vi "To Dynamic Signal.vi"(8 "error in (no error)":errorcluster, 11 "Software Lock-in in":refnum<class "Software Lock-in.lvclass">) -> (0 "error out":errorcluster, 1 "Channel names":string[](array[string]), 2 "Signal":dynamicdata(graph), 3 "Software Lock-in out":refnum<class "Software Lock-in.lvclass">, 4 "Time axis":dbl[](array[numeric]), 5 "dt":dbl)   [LabVIEW 2016, in "Software Lock-in.lvclass"]
uses:
  Software Lock-in.lvclass
  Software Lock-in.lvclass/Software Lock-in.ctl
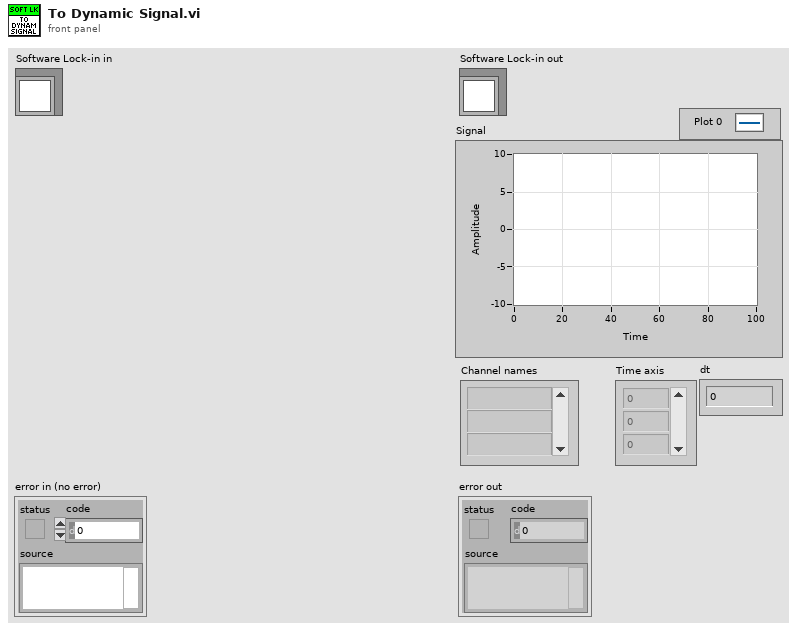
[diagram p1: front panel]
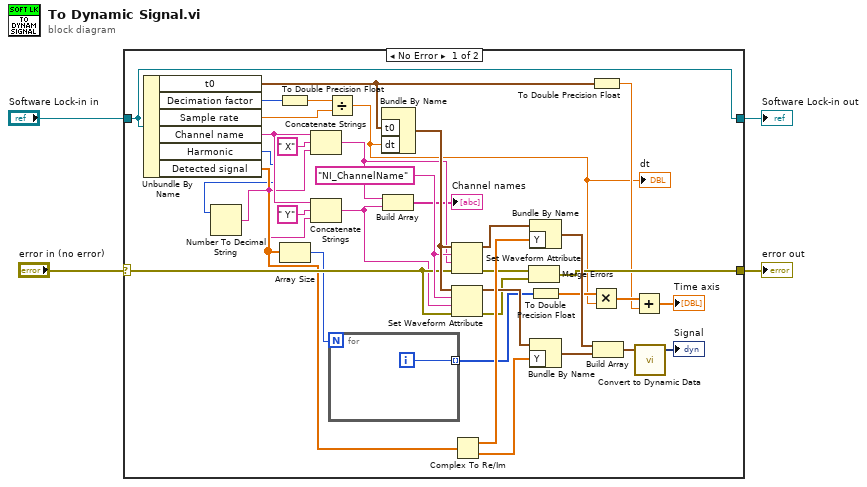
[diagram p0: block diagram]
diagram:
  n1 = case shown="No Error" "error in (no error)" {
    selector: "error in (no error)" -> [w20 w42]
    tunnel: [w19 w42] -> w3
    tunnel: [w39 w41] -> w1
    tunnel: "Software Lock-in in" -> [w39 w41]
    frame No Error {
      w33 = "NI_ChannelName" ("Channel Name")
      n2 = Unbundle By Name(w39) -> ("t0"=w10:timestamp, "Decimation factor"=w38:i32, "Sample rate"=w36:dbl, "Channel name"=w31:string, "Harmonic"=w6:i32, "Detected signal"=w15:cdb[])
      n3 = Number To Decimal String(number=w6) -> (decimal integer string=w5:string)  [unwired: 1 in]
      n4 = To Double Precision Float(number=w38) -> (double precision float=w37:dbl)
      n5 = Array Size(array=w15) -> (size(s)=w14:i32)
      n6 = Concatenate Strings(w31, " X" ("string"), w5) -> (w18:string)
      n7 = Concatenate Strings(w31, " Y" ("string"), w5) -> (w17:string)
      n8 = Divide(x=w37, y=w36) -> (x/y=w7:dbl)
      "dt" <- w7
      n9 = for {
        N: w14 -> [_]
        tunnel: [w40] -> w13 mode=indexing
        i -> [w40]
      }
      n10 = Bundle By Name("t0"=w10, "dt"=w7) -> (w34:waveform(dbl))  [unwired: 1 in]
      n11 = Build Array(w18, w17) -> (→"Channel names":string[])
      n12 = Set Waveform Attribute(4:w20, 5:w18, 6:w33, 7:w34) -> (0:w22:errorcluster, 3:w30:waveform(dbl))  [unwired: 1 out]
      n13 = Set Waveform Attribute(4:w20, 5:w17, 6:w33, 7:w34) -> (0:w21:errorcluster, 3:w28:waveform(dbl))  [unwired: 1 out]
      n14 = Complex To Re/Im(x + iy=w15) -> (x=w29:dbl[], y=w27:dbl[])
      n15 = Merge Errors(w22, w21) -> (w19:errorcluster)
      n16 = Bundle By Name(cluster=w30, "Y"=w29) -> (w26:waveform(dbl))
      n17 = Bundle By Name(cluster=w28, "Y"=w27) -> (w25:waveform(dbl))
      n18 = To Double Precision Float(number=w13) -> (double precision float=w12:dbl[])
      n19 = Multiply(x=w12, y=w7) -> (x*y=w11:dbl[])
      n20 = To Double Precision Float(number=w10) -> (double precision float=w9:dbl)
      n21 = Build Array(w26, w25) -> (w24:waveform(dbl)[])
      n22 = Add(x=w11, y=w9) -> (x+y=→"Time axis":dbl[])
      n23 = call "Convert to Dynamic Data"("Array of Waveforms"=w24) -> ("Dynamic Data Type"=→"Signal":dynamicdata)  [unwired: 3 in]
    }
    frame Error {
    }
  }
  "error out" <- w3
  "Software Lock-in out" <- w1
